vi "Is Site in Map.vi"(8 "error in":errorcluster, 10 "site":i32, 11 "connection map in":refnum<class "Connection Map.lvclass">) -> (0 "error out":errorcluster, 2 "site in map":bool, 3 "connection map out":refnum<class "Connection Map.lvclass">)   [LabVIEW 2020, in "Plug-In SDK Session Management V1 API.lvlib" / "Connection Map.lvclass"]
uses:
  Connection Map.lvclass
  d9ff3614-c2db-4564-ba54-f6f8c522c897.vi
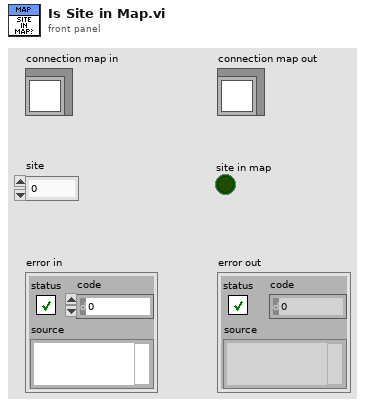
[diagram p1: front panel]
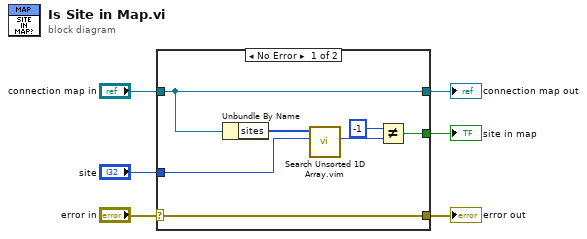
[diagram p0: block diagram]
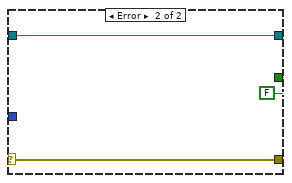
[diagram p2: hidden frame]
diagram:
  n1 = case shown="No Error" "error in" {
    selector: "error in" -> [w13 w16]
    tunnel: [w13 w16] -> w5
    tunnel: [w12 w15] -> w3
    tunnel: "connection map in" -> [w12 w15]
    tunnel: "site" -> [w8 _]
    tunnel: [w7 FALSE ("key not found?")] -> w1
    frame No Error {
      n2 = Unbundle By Name(w12) -> ("sites"=w9:i32[])
      n3 = call "Search Unsorted 1D Array.vim"("element"=w8, "unsorted 1D array"=w9) -> ("index of element"=w11:i32)  [unwired: 9 in]
      n4 = Not Equal?(x=-1, y=w11) -> (x != y?=w7:bool)
    }
    frame Error {
    }
  }
  "error out" <- w5
  "connection map out" <- w3
  "site in map" <- w1
